vi "DAC Run.vi"(8 "error in":errorcluster, 11 "DAC Vacum Pressure in":refnum<class "DAC Vacum Pressure.lvclass">) -> (0 "error out":errorcluster, 3 "DAC Vacum Pressure out":refnum<class "DAC Vacum Pressure.lvclass">)   [LabVIEW 2019, in "DAC.lvlib" / "DAC Vacum Pressure.lvclass"]
uses:
  DAC Vacum Pressure.lvclass
  DAC.lvclass
  Results/Results Method.ctl
  Results/Results.lvlib
  Results/HTS Results/HTS Results.lvclass
  <vilib>/ErrorRing/Error Ring.xnode
  <vilib>/Utility/error.llb/Error Cluster From Error Code.vi
  <vilib>/DAQmx/read.llb/DAQmx Read (Analog DBL 1Chan 1Samp).vi
  C:/Users/krio/Documents/LV_Projects/test-stand/App/DAC/DAC.lvclass
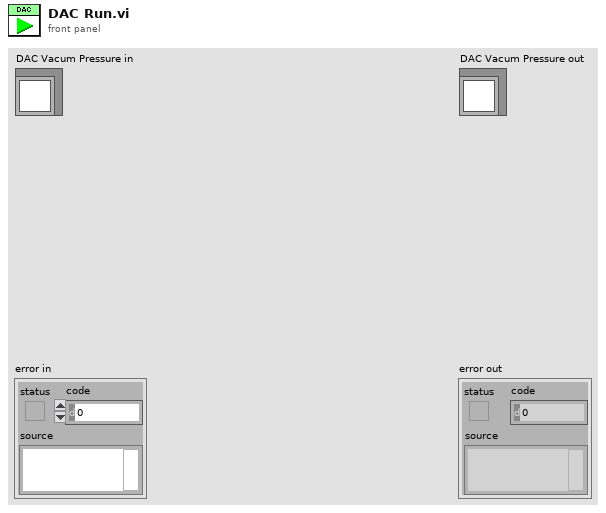
[diagram p1: front panel]
types:
  T1 = typedef "Results.lvlib/Results Method.ctl" = enum16{"Get", "Set"}
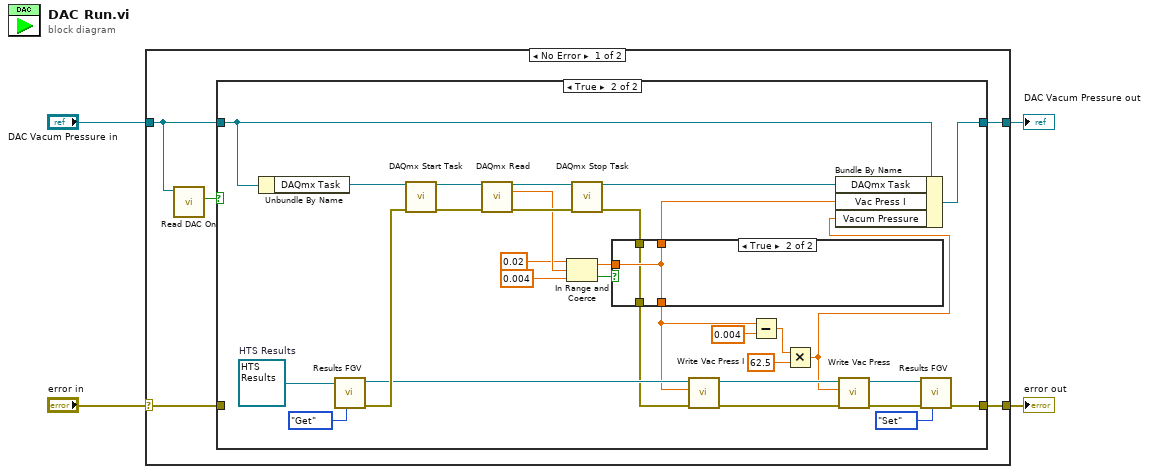
[diagram p0: block diagram]
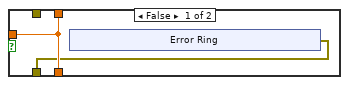
[diagram p3: hidden frame]
diagram:
  n1 = case shown="No Error" "error in" {
    selector: "error in" -> [w7 w52]
    tunnel: [w6 w52] -> w2
    tunnel: [w8 w51] -> w1
    tunnel: "DAC Vacum Pressure in" -> [w5 w51]
    frame No Error {
      n2 = call "Read DAC On.vi"("DAC in"=w5) -> ("DAC On"=w9:bool)  [unwired: 8 in, 2 out]
      n3 = case shown="True" w9 {
        tunnel: w5 -> [w11 w38]
        tunnel: [w11 w31] -> w8
        tunnel: w7 -> [w10 _]
        tunnel: [w10 w30] -> w6
        frame False {
        }
        frame True {
          w37 = refnum<class "HTS Results.lvclass"> refnum  # HTS Results
          n4 = Unbundle By Name(w38) -> ("DAQmx Task"=w42:refnum<k21>)
          n5 = call-dynamic "Results FGV.vi"("Method"=Results_Method."Get", "HTS Results in"=w37) -> ("error out"=w34:errorcluster, "HTS Results out"=w18:refnum<class "HTS Results.lvclass">)  [unwired: 8 in]
          n6 = call <vilib>:"DAQmx Start Task.vi"("task/channels in"=w42, "error in"=w34) -> ("task out"=w41:refnum<k21>, "error out"=w40:errorcluster)  [unwired: 12 in]
          n7 = call-poly <vilib>:"DAQmx Read.vi"("task/channels in"=w41, "error in"=w40) -> ("task out"=w32:refnum<k21>, "data"=w29:dbl, "error out"=w39:errorcluster)  [unwired: 11 in]
          n8 = In Range and Coerce(upper limit=0.02, x=w29, lower limit=0.004) -> (coerced(x)=w27:dbl, In Range?=w28:bool)
          n9 = call <vilib>:"DAQmx Stop Task.vi"("task/channels in"=w32, "error in"=w39) -> ("task out"=w33:refnum<k21>, "error out"=w16:errorcluster)  [unwired: 12 in]
          n10 = case shown="True" w28 {
            tunnel: w27 -> [w44 w50]
            tunnel: [w44 w50] -> w12
            tunnel: [w44 w50] -> w21
            tunnel: w16 -> [_ w49]
            tunnel: [w43 w49] -> w15
            frame False {
              n11 = xnode "Error Ring"() -> ("error out"=w43:errorcluster)
            }
            frame True {
            }
          }
          n12 = call "Write Vac Press I.vi"("error in (no error)"=w15, "Vac Press I"=w12, "HTS Results in"=w18) -> ("error out"=w14:errorcluster, "HTS Results out"=w17:refnum<class "HTS Results.lvclass">)  [unwired: 7 in]
          n13 = Subtract(x=w12, y=0.004) -> (x-y=w23:dbl)
          n14 = Multiply(x=w23, y=62.5) -> (x*y=w13:dbl)
          n15 = Bundle By Name(cluster=w38, "DAQmx Task"=w33, "Vac Press I"=w21, "Vacum Pressure"=w13) -> (w31:refnum<class "DAC Vacum Pressure.lvclass">)
          n16 = call "Write Vac Press.vi"("error in (no error)"=w14, "Vac Press"=w13, "HTS Results in"=w17) -> ("error out"=w19:errorcluster, "HTS Results out"=w20:refnum<class "HTS Results.lvclass">)  [unwired: 7 in]
          n17 = call-dynamic "Results FGV.vi"("Method"=Results_Method."Set", "error in"=w19, "HTS Results in"=w20) -> ("error out"=w30:errorcluster)  [unwired: 7 in, 1 out]
        }
      }
    }
    frame Error {
    }
  }
  "error out" <- w2
  "DAC Vacum Pressure out" <- w1
